vi "GetFrameFaultInfo.vi"(5 "XNET Cluster":refnum<k21>, 7 "Frame Array":string[](array[string]), 8 "error in (no error)":errorcluster, 9 "Frame Direction":T1, 10 "ECU Reference":refnum<k21>, 11 "Device Item Ref in":T2 format="%.0x") -> (0 "error out":errorcluster, 2 "Array":T3[](array[typedef]) {"CRC Index" min=-7 max=7; "DLC Length  Corruption Index" min=-7 max=7}, 3 "Frame ID Array":u32[](array[numeric]))   [LabVIEW 2018, in "CAN Gateway System Explorer.lvlib"]
uses:
  CAN Gateway System Explorer.lvlib
  Shared/CTLs/Frame.ctl
  Shared/CTLs/Signal_Data_Trigger.ctl
  <vilib>/NI Veristand/Custom Device API/Custom Device Item Ref.ctl
  Types/FrameDirection.ctl
  Shared/Constants.vi
  <vilib>/NI Veristand/Custom Device API/Get Item Property (Boolean).vi
  <vilib>/NI Veristand/Custom Device Tools/Custom Device Utility Library/NI VeriStand - Search for Item by Name.vi
  <vilib>/NI Veristand/Custom Device API/Custom Device API.lvlib
  Shared/CAN Gateway Shared.lvlib
  <resource>/objmgr/xnet.rc
  <vilib>/NI Veristand/Custom Device Tools/Custom Device Utility Library/Custom Device Utility Library.lvlib
panel:
  in  "Empty?":bool
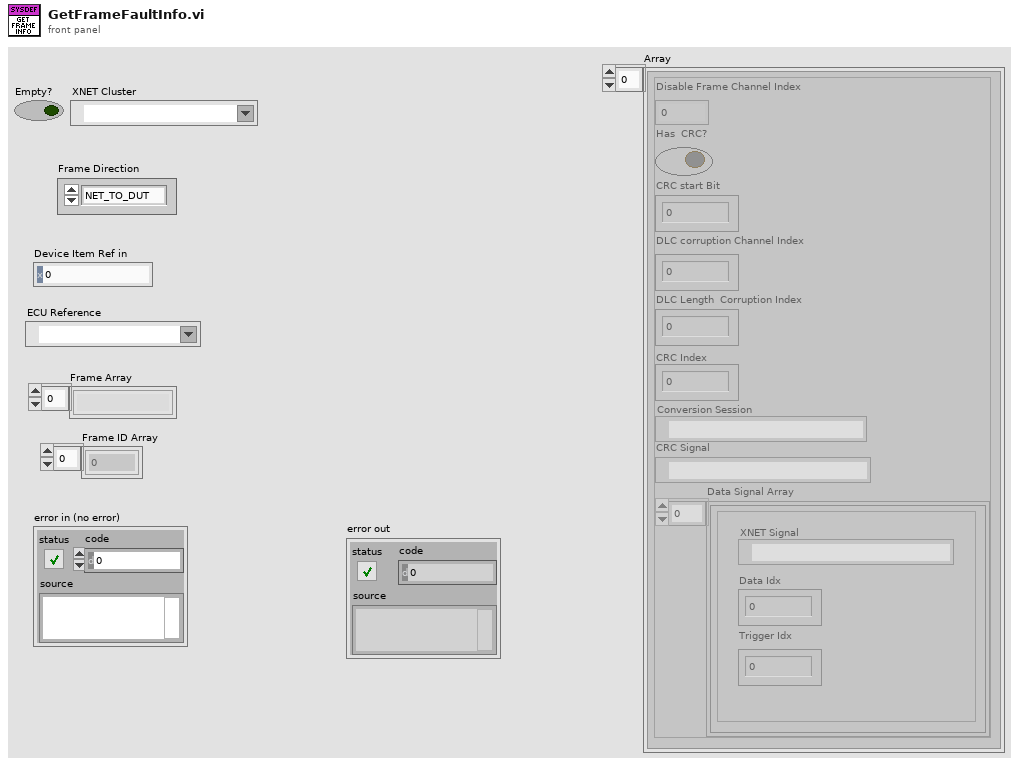
[diagram p1: front panel]
types:
  T1 = typedef "CAN Gateway System Explorer.lvlib/FrameDirection.ctl" = enum16{"NET_TO_DUT", "DUT_TO_NET"}
  T2 = typedef "Custom Device API.lvlib/Custom Device Item Ref.ctl" = u64
  T3 = typedef "CAN Gateway Shared.lvlib/Frame.ctl" = cluster{"Disable Frame Channel Index":i32, "Has  CRC?":bool, "CRC start Bit":u32, "DLC corruption Channel Index":i32, "DLC Length  Corruption Index":i32, "CRC Index":i32, "Conversion Session":refnum<k21>, "CRC Signal":refnum<k21>, "Data Signal Array":T4[]}
  T4 = typedef "CAN Gateway Shared.lvlib/Signal_Data_Trigger.ctl" = cluster{"XNET Signal":refnum<k21>, "Data Idx":u32, "Trigger Idx":u32}
  T5 = typedef "Custom Device API.lvlib/Custom Device Item Info.ctl" = cluster{"Name":string, "Is Channel":bool, "GUID":string, "Is Waveform":bool}
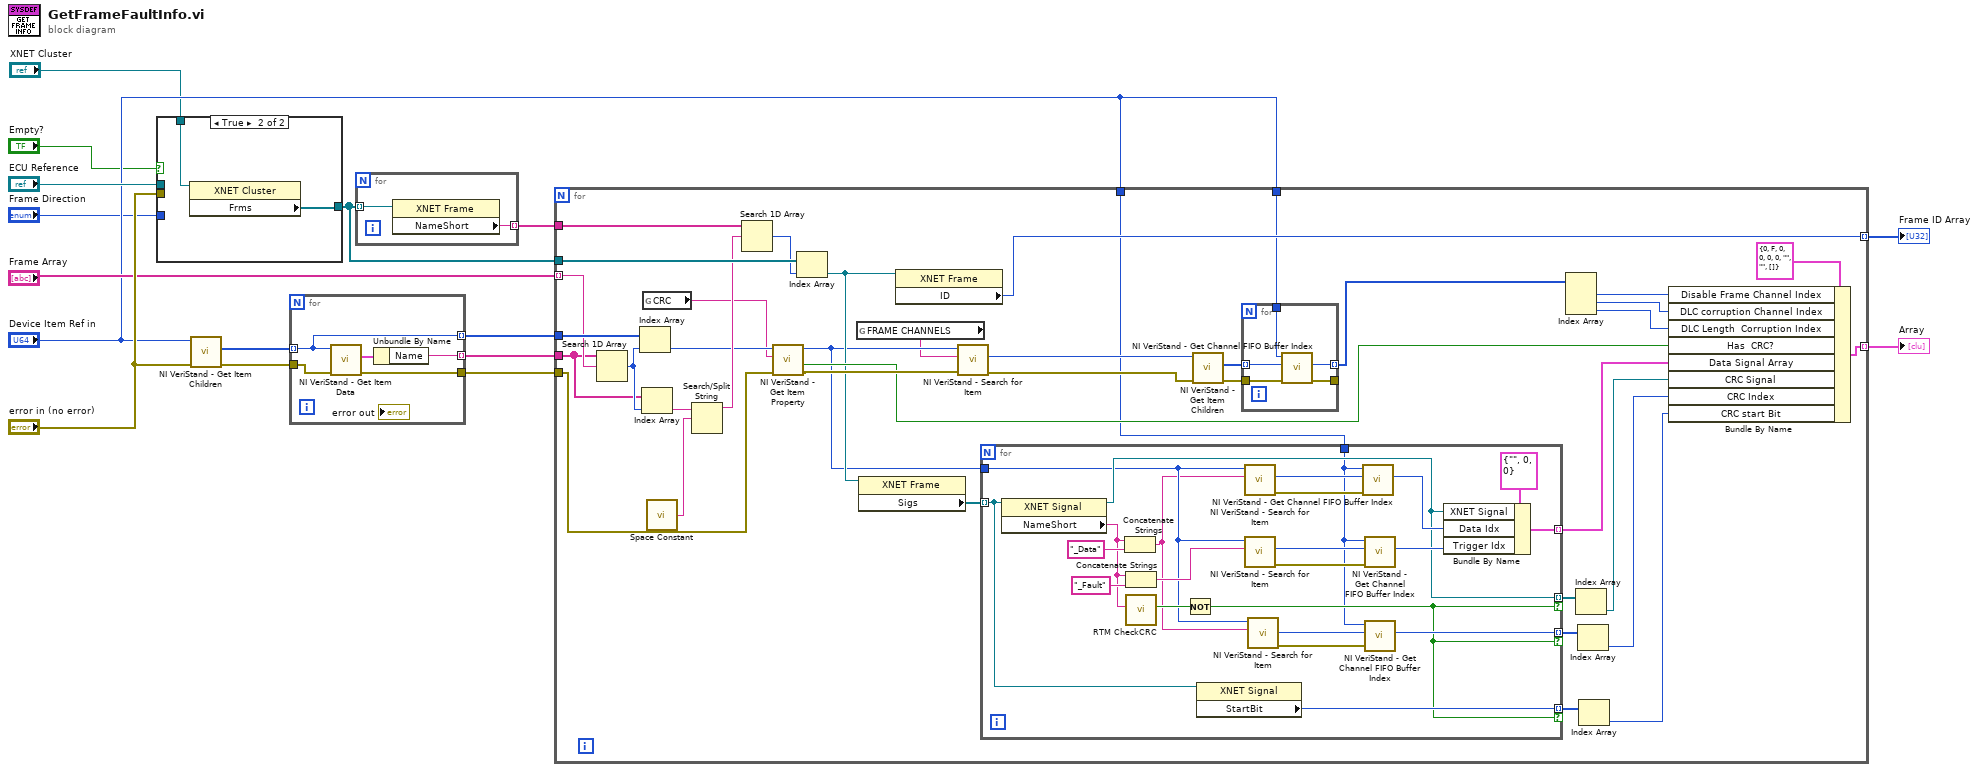
[diagram p0: block diagram]
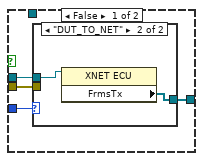
[diagram p2: hidden frame]
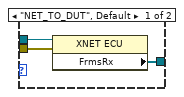
[diagram p3: hidden frame]
diagram:
  n1 = case shown="True" "Empty?" {
    tunnel: [w20 w26] -> w14
    tunnel: "error in (no error)" -> [w19 _]
    tunnel: "ECU Reference" -> [w18 _]
    tunnel: "Frame Direction" -> [w17 _]
    tunnel: "XNET Cluster" -> [_ w27]
    frame False {
      n2 = case shown="\"DUT_TO_NET\"" w17 {
        tunnel: [w23 w25] -> w20
        tunnel: w19 -> [w22 _]
        tunnel: w18 -> [w21 w24]
        frame "NET_TO_DUT", Default {
          n3 = property class="XNET ECU"(reference=w21, error in=w22) -> ("FrmsRx"=w23:refnum<k21>[])  [unwired: 2 out]
        }
        frame "DUT_TO_NET" {
          n4 = property class="XNET ECU"(reference=w24) -> ("FrmsTx"=w25:refnum<k21>[])  [unwired: 1 in, 2 out]
        }
      }
    }
    frame True {
      n5 = property class="XNET Cluster"(reference=w27) -> ("Frms"=w26:refnum<k21>[])  [unwired: 1 in, 2 out]
    }
  }
  n6 = call <vilib>:"NI VeriStand - Get Item Children.vi"("error in (no error)"="error in (no error)", "Item Ref in"="Device Item Ref in") -> ("error out"=w8:errorcluster, "Child Refs"=w7:T2[])  [unwired: 6 in, 2 out]
  n7 = for {
    tunnel: w7 -> [w28] mode=indexing
    tunnel: w8 -> [w31]
    tunnel: [w30] -> w6
    tunnel: [w29] -> w9 mode=indexing
    tunnel: [w28] -> w10 mode=indexing
    n8 = call <vilib>:"NI VeriStand - Get Item Data.vi"("error in (no error)"=w31, "Item Ref in"=w28) -> ("error out"=w30:errorcluster, "Item Info"=w32:T5)  [unwired: 6 in, 2 out]
    n9 = Unbundle By Name(w32) -> ("Name"=w29:string)
  }
  n10 = for {
    tunnel: w14 -> [w34] mode=indexing
    tunnel: [w33] -> w15 mode=indexing
    n11 = property class="XNET Frame"(reference=w34) -> ("NameShort"=w33:string)  [unwired: 1 in, 2 out]
  }
  n12 = for {
    tunnel: w9 -> [w70]
    tunnel: w10 -> [w73]
    tunnel: "Frame Array" -> [w72] mode=indexing
    tunnel: w14 -> [w66]
    tunnel: w15 -> [w67]
    tunnel: [w63] -> w16 mode=indexing
    tunnel: w6 -> [w49]
    tunnel: "Device Item Ref in" -> [w59]
    tunnel: "Device Item Ref in" -> [w44]
    tunnel: [w43] -> w4 mode=indexing
    n13 = Search 1D Array(1D array=w70, element=w72) -> (index of element=w71:i32)  [unwired: 1 in]
    n14 = Index Array(array=w73, index=w71) -> (element=w52:T2)
    n15 = Index Array(array=w70, index=w71) -> (element=w69:string)
    n16 = global read "Constants.vi" "CRC"() -> (w50:string)
    n17 = call <vilib>:"Space Constant.vi"() -> ("String"=w68:string)
    n18 = Search/Split String(string=w69, search string/char (-)=w68) -> (substring before match=w64:string)  [unwired: 1 in, 2 out]
    n19 = Search 1D Array(1D array=w67, element=w64) -> (index of element=w65:i32)  [unwired: 1 in]
    n20 = call-poly <vilib>:"NI VeriStand - Get Item Property.vi"("error in (no error)"=w49, "Property Name"=w50, "Item Ref in"=w52) -> ("error out"=w51:errorcluster, "Value"=w48:bool, "Item Ref out"=w45:T2)  [unwired: 5 in, 1 out]
    n21 = Index Array(array=w66, index=w65) -> (element=w47:refnum<k21>)
    n22 = global read "Constants.vi" "FRAME CHANNELS"() -> (w38:string)
    n23 = property class="XNET Frame"(reference=w47) -> ("Sigs"=w46:refnum<k21>[])  [unwired: 1 in, 2 out]
    n24 = property class="XNET Frame"(reference=w47) -> ("ID"=w63:u32)  [unwired: 1 in, 2 out]
    n25 = call-poly <vilib>:"NI VeriStand - Search for Item.vi"("error in"=w51, "Item Name"=w38, "Section Ref in"=w45) -> ("error out"=w61:errorcluster, "Item Ref"=w62:T2)  [unwired: 5 in, 2 out]
    n26 = for {
      tunnel: w46 -> [w83] mode=indexing
      tunnel: w45 -> [w80]
      tunnel: w44 -> [w75]
      tunnel: [w86] -> w40 mode=indexing
      tunnel: [w84] -> w42 mode=indexing if=w76
      tunnel: [w82] -> w41 mode=indexing if=w76
      tunnel: [w77] -> w37 mode=indexing if=w76
      n27 = property class="XNET Signal"(reference=w83) -> (reference out=w84:refnum<k21>, "NameShort"=w85:string)  [unwired: 1 in, 1 out]
      n28 = Concatenate Strings(w85, "_Data" ("Item Name")) -> (w79:string)
      n29 = Concatenate Strings(w85, "_Fault" ("Item Name")) -> (w94:string)
      n30 = call "RTM CheckCRC.vi"("SignalName"=w85) -> ("CRC?"=w81:bool)  [unwired: 8 in, 2 out]
      n31 = Not(x=w81) -> (.not. x?=w76:bool)
      n32 = property class="XNET Signal"(reference=w83) -> ("StartBit"=w82:u32)  [unwired: 1 in, 2 out]
      n33 = call-poly <vilib>:"NI VeriStand - Search for Item.vi"("Item Name"=w79, "Section Ref in"=w80) -> ("error out"=w92:errorcluster, "Item Ref"=w93:T2)  [unwired: 6 in, 2 out]
      n34 = call-poly <vilib>:"NI VeriStand - Search for Item.vi"("Item Name"=w94, "Section Ref in"=w80) -> ("error out"=w91:errorcluster, "Item Ref"=w90:T2)  [unwired: 6 in, 2 out]
      n35 = call-poly <vilib>:"NI VeriStand - Search for Item.vi"("Item Name"=w79, "Section Ref in"=w80) -> ("error out"=w78:errorcluster, "Item Ref"=w74:T2)  [unwired: 6 in, 2 out]
      n36 = call <vilib>:"NI VeriStand - Get Channel FIFO Buffer Index.vi"("error in"=w92, "Channel Ref"=w93, "Device Ref in"=w75) -> ("Channel FIFO Buffer Index"=w88:i32)  [unwired: 4 in, 4 out]
      n37 = call <vilib>:"NI VeriStand - Get Channel FIFO Buffer Index.vi"("error in"=w91, "Channel Ref"=w90, "Device Ref in"=w75) -> ("Channel FIFO Buffer Index"=w87:i32)  [unwired: 4 in, 4 out]
      n38 = call <vilib>:"NI VeriStand - Get Channel FIFO Buffer Index.vi"("error in"=w78, "Channel Ref"=w74, "Device Ref in"=w75) -> ("Channel FIFO Buffer Index"=w77:i32)  [unwired: 4 in, 4 out]
      n39 = Bundle By Name(cluster=T4 {"XNET Signal"="", "Data Idx"=0, "Trigger Idx"=0} ("Signal Data Trigger"), "XNET Signal"=w84, "Data Idx"=w88, "Trigger Idx"=w87) -> (w86:T4)
    }
    n40 = call <vilib>:"NI VeriStand - Get Item Children.vi"("error in (no error)"=w61, "Item Ref in"=w62) -> ("error out"=w57:errorcluster, "Child Refs"=w58:T2[])  [unwired: 6 in, 2 out]
    n41 = for {
      tunnel: w59 -> [w101]
      tunnel: w58 -> [w100] mode=indexing
      tunnel: w57 -> [w99]
      tunnel: [w98] -> _
      tunnel: [w97] -> w56 mode=indexing
      n42 = call <vilib>:"NI VeriStand - Get Channel FIFO Buffer Index.vi"("error in"=w99, "Channel Ref"=w100, "Device Ref in"=w101) -> ("error out"=w98:errorcluster, "Channel FIFO Buffer Index"=w97:i32)  [unwired: 4 in, 3 out]
    }
    n43 = Index Array(array=w56) -> (element #1=w55:i32, element #2=w54:i32, element #3=w53:i32)  [unwired: 3 in]
    n44 = Index Array(array=w42) -> (element=w39:refnum<k21>)  [unwired: 1 in]
    n45 = Index Array(array=w37) -> (element=w36:i32)  [unwired: 1 in]
    n46 = Index Array(array=w41) -> (element=w35:u32)  [unwired: 1 in]
    n47 = Bundle By Name(cluster=T3 {"Disable Frame Channel Index"=0, "Has  CRC?"=FALSE, "CRC start Bit"=0, "DLC corruption Channel Index"=0, "DLC Length  Corruption Index"=0, "CRC Index"=0, "Conversion Session"="", "CRC Signal"="", "Data Signal Array"=[]} ("Frame Infos"), "Disable Frame Channel Index"=w55, "DLC corruption Channel Index"=w54, "DLC Length  Corruption Index"=w53, "Has  CRC?"=w48, "Data Signal Array"=w40, "CRC Signal"=w39, "CRC Index"=w36, "CRC start Bit"=w35) -> (w43:T3)
  }
  "Array" <- w4
  "Frame ID Array" <- w16
